vi "Review Fiducials Dialog.vi"(7 "Console Log in":refnum<class "Console Log.lvclass">, 8 "error in":errorcluster, 11 "Potting Procedure in":refnum<class "Potting Procedure.lvclass">) -> (0 "error out":errorcluster, 2 "Canceled":bool, 3 "Potting Procedure out":refnum<class "Potting Procedure.lvclass">, 5 "Console Log out":refnum<class "Console Log.lvclass">)   [LabVIEW 2011]
uses:
  Procedure Classes/Potting Procedure/Potting Procedure.lvclass
  UI Classes/Console Log/Console Log.lvclass
  Shared Components/Utils/Type Definitions/Fiducial with Source.ctl
  Shared Components/Vec3d Class/Vec3d Class.lvclass
  Procedure Classes/Potting Procedure/Type Definitions/Inspect Fiducials.ctl
  Shared Components/Utils/Type Definitions/Fiducial Image.ctl
  Shared Components/Utils/Type Definitions/Physical Image.ctl
  <vilib>/vision/Image Controls.llb/IMAQ Image.ctl
  Procedure Classes/Potting Procedure/Type Definitions/Review Fiducials.ctl
panel:
  out "BBM BL View":T1(plugin-control)
  out "BBM BR View":T1(plugin-control)
  out "BBM TL View":T1(plugin-control)
  out "BBM TR View":T1(plugin-control)
  in  "idx":i32
  out "idx_label":string="1/10"
  out "Current Module":cluster{"Chuck":i32, "Slot":i32}={"Chuck"=1, "Slot"=1}
  in  "Previous":bool
  in  "Next":bool
  out "HDI BL View":T1(plugin-control)
  out "HDI BR View":T1(plugin-control)
  out "HDI TL View":T1(plugin-control)
  out "HDI TR View":T1(plugin-control)
  in  "OK Button":bool
  in  "Cancel Button":bool
  # "Pattern Recognition"
  # "Error"
  # "Click on images to correct fiducial positions.\nAll error fiducials must be corrected before continuing."
  # "User Defined"
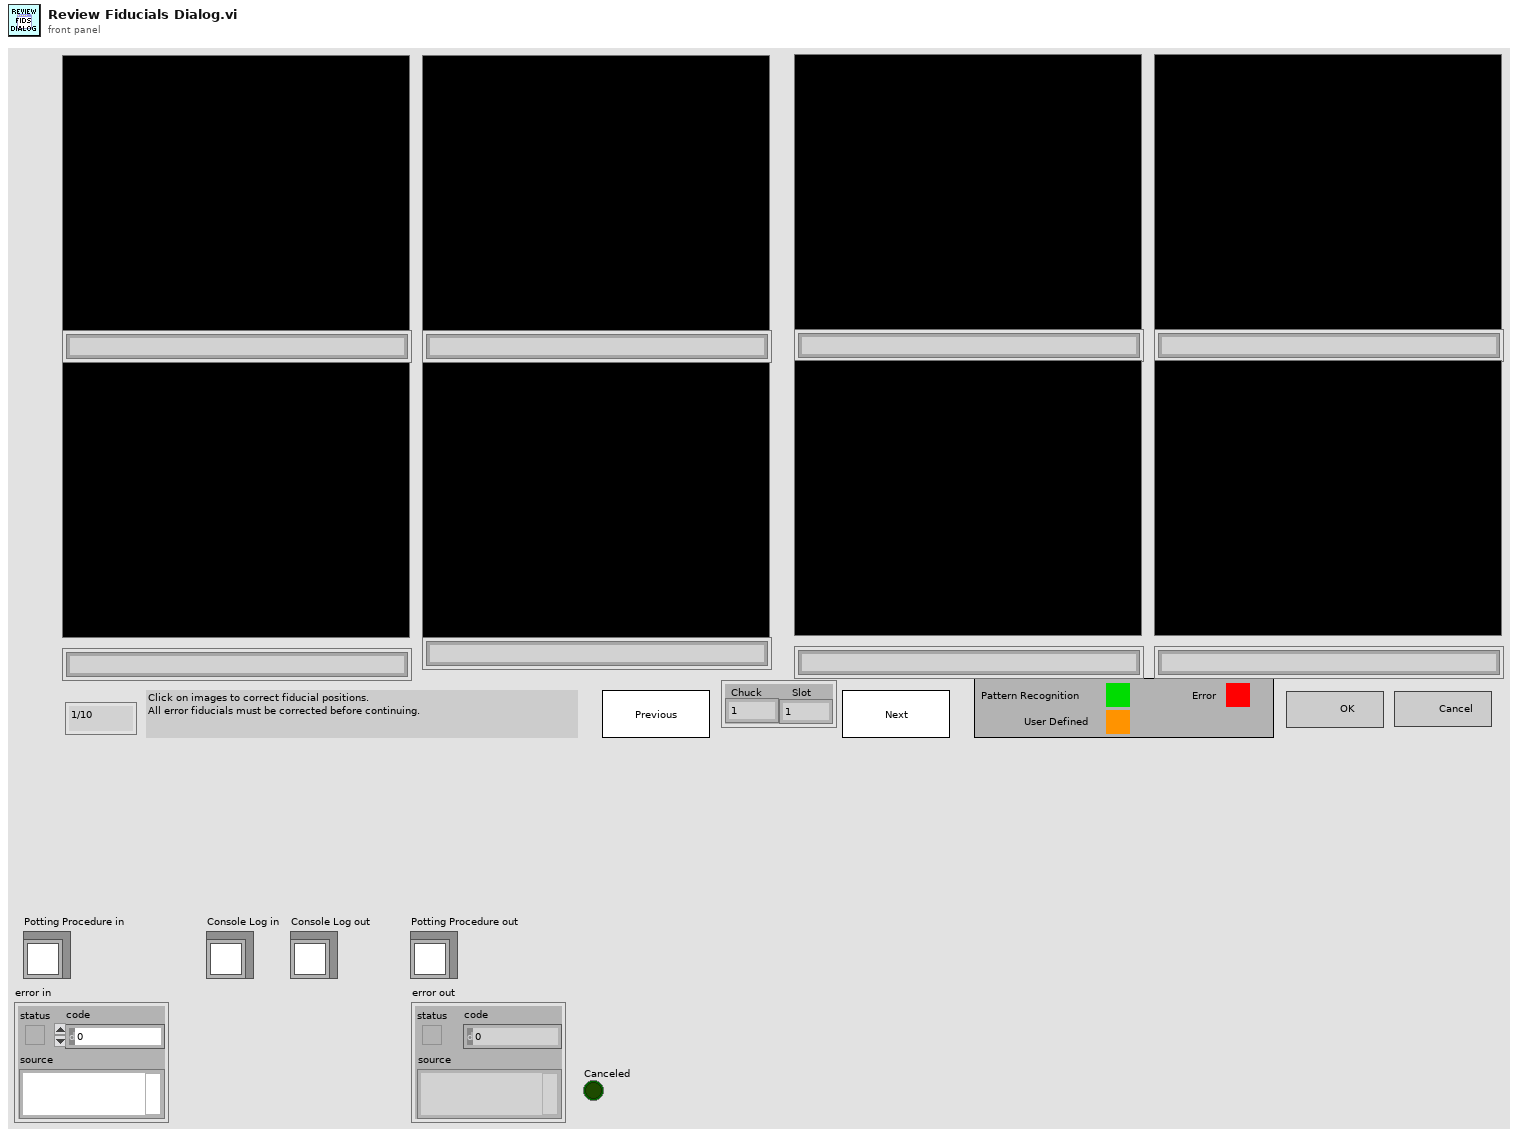
[diagram p1: front panel]
types:
  T1 = typedef "IMAQ Image.ctl" = refnum<image>
  T2 = typedef "Inspect Fiducials.ctl" = cluster{"Has Been Run?":bool, "Module-Chuck Fiducials":cluster{"Fiducials-HDI":T3[], "Fiducials-BBM":T3[], "Chuck":i32, "Slot":i32}[]}
  T3 = typedef "Fiducial Image.ctl" = cluster{"Fiducial Image":T4, "Selected Fiducial":T5, "fiducial name":string}
  T4 = typedef "Physical Image.ctl" = cluster{"Image Position":refnum<class "Vec3d Class.lvclass">, "Image Reference":T1, "Field of View":cluster{"x(mm)":dbl, "y(mm)":dbl}}
  T5 = typedef "Fiducial with Source.ctl" = cluster{"Fiducial Image Coordinate":refnum<class "Vec3d Class.lvclass">, "Fiducial Source":enum16{"Pattern Recognition", "User", "Error", "Default"}}
  T6 = cluster{"Fiducials-HDI":T3[], "Fiducials-BBM":T3[], "Chuck":i32, "Slot":i32}[]
  T7 = cluster{"Fiducials-HDI":T3[], "Fiducials-BBM":T3[], "Chuck":i32, "Slot":i32}
  T8 = enum16{"Pattern Recognition", "User", "Error", "Default"}
  T9 = typedef "LVPoint32TypeDef.ctl" = cluster{"Horizontal":i32, "Vertical":i32}
  T10 = typedef "Review Fiducials.ctl" = cluster{"Has Been Run?":bool}
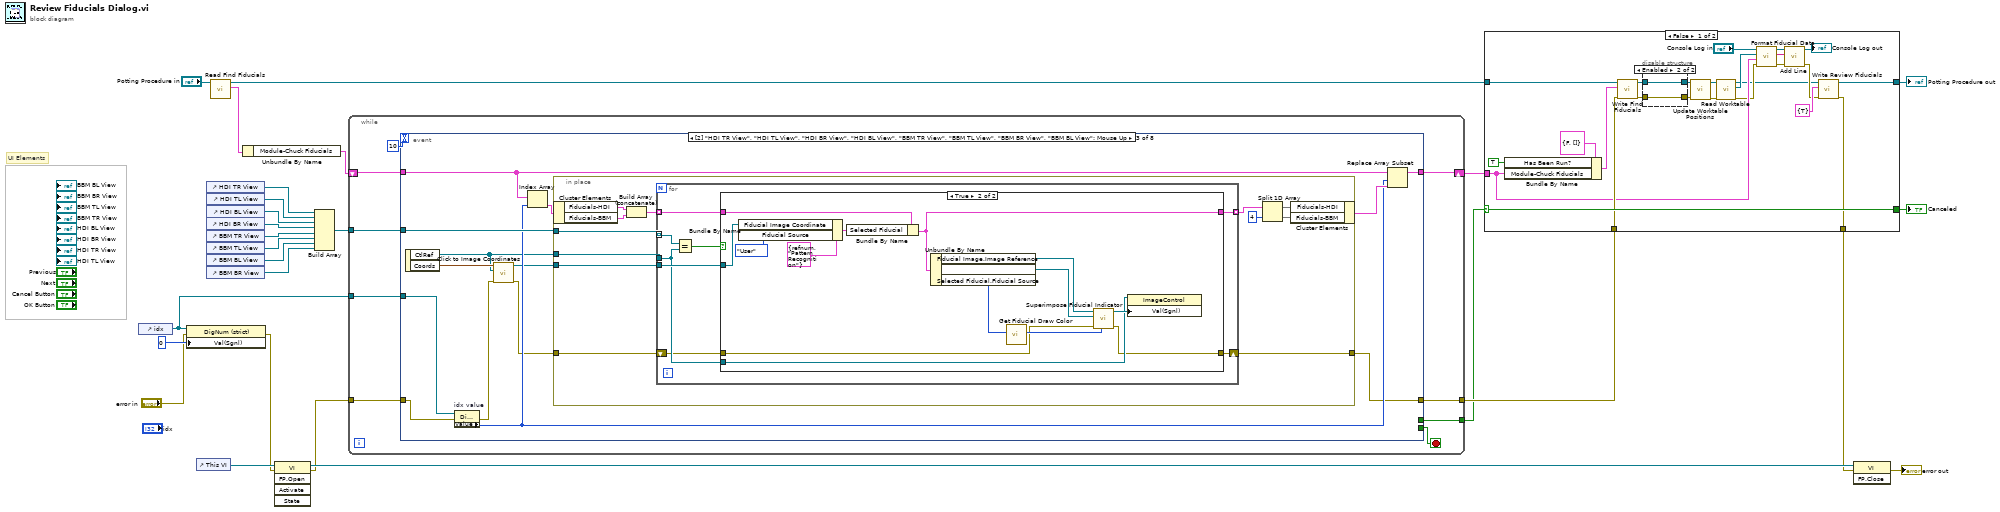
[diagram p0: block diagram]
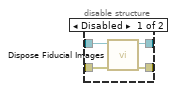
[diagram p2: hidden frame]
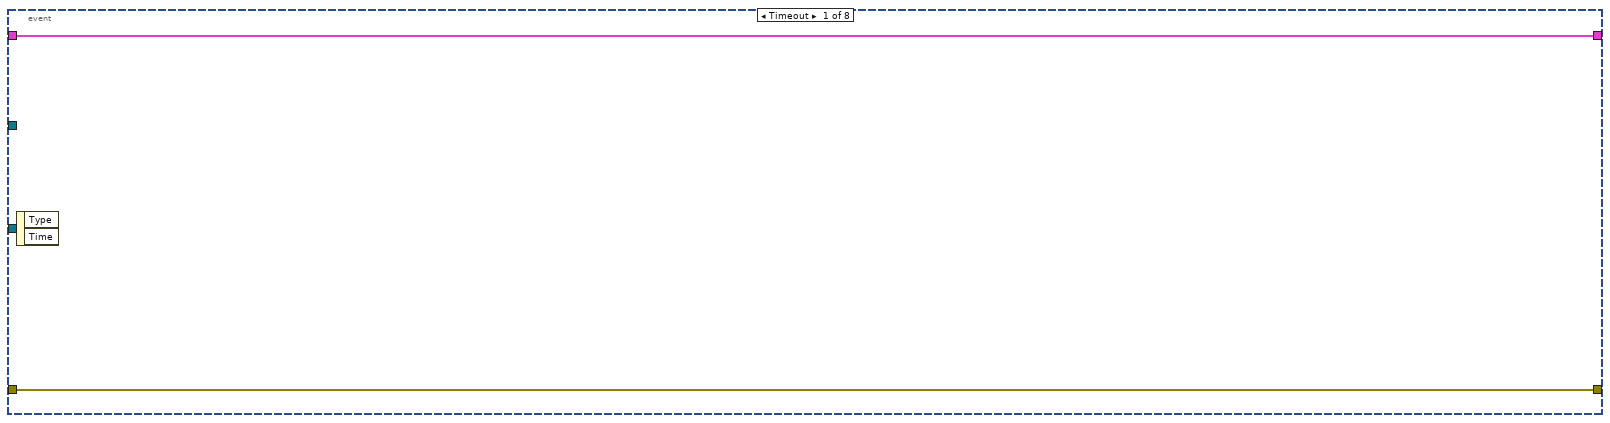
[diagram p4: hidden frame]
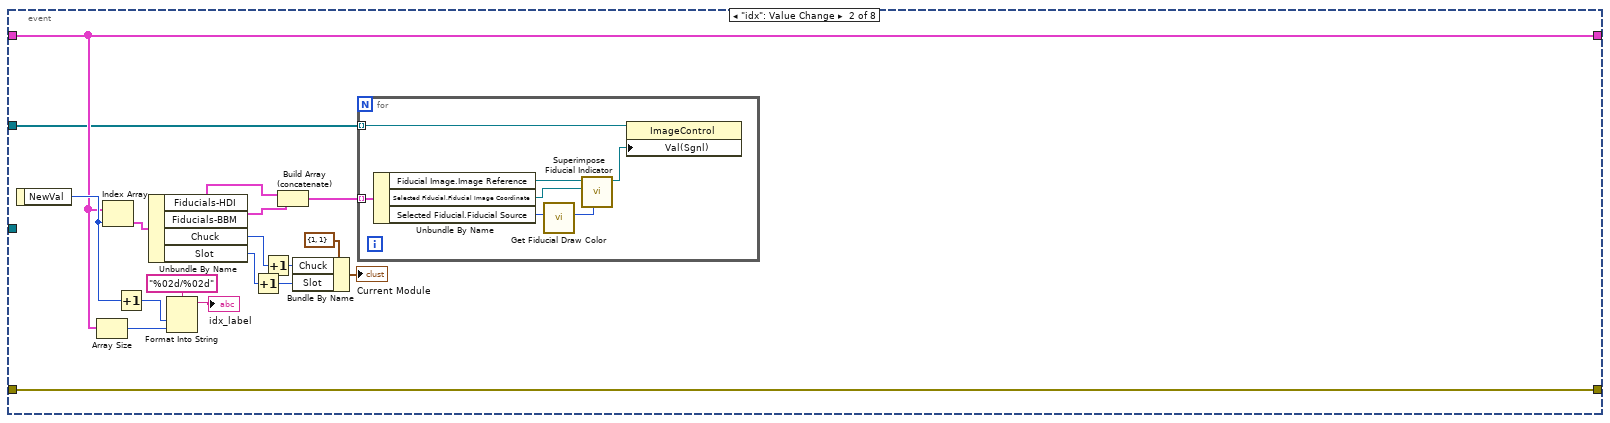
[diagram p5: hidden frame]
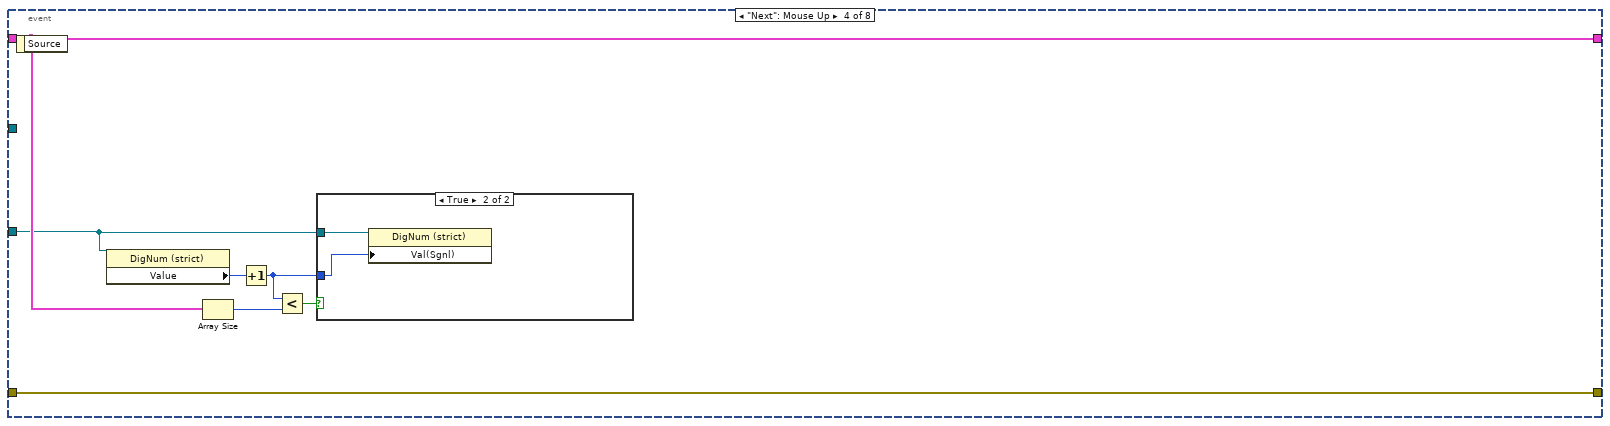
[diagram p7: hidden frame]
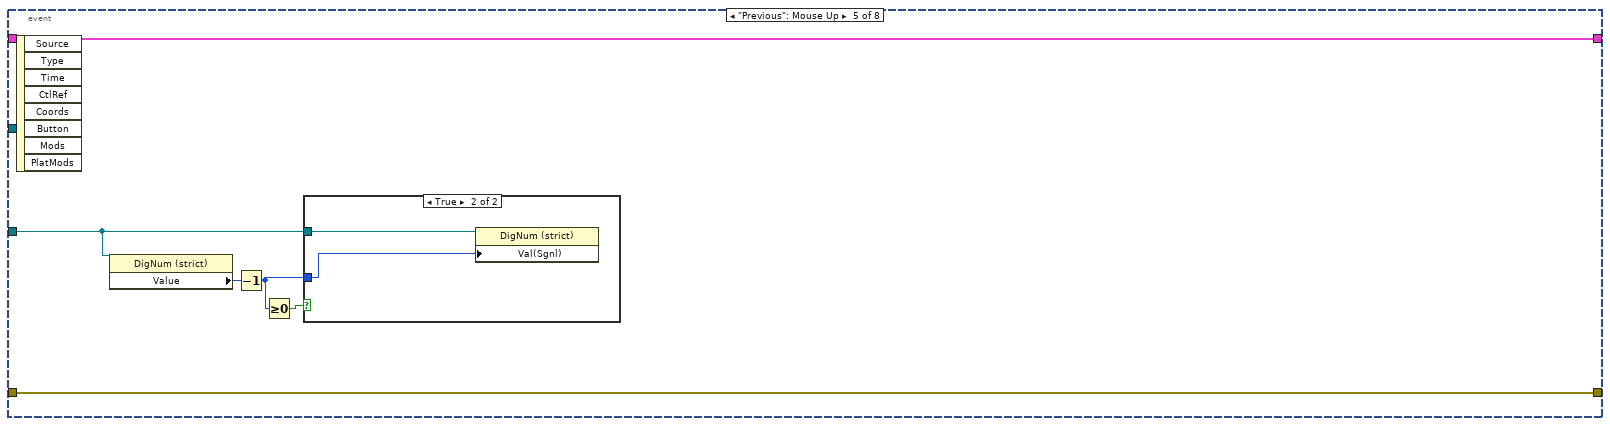
[diagram p9: hidden frame]
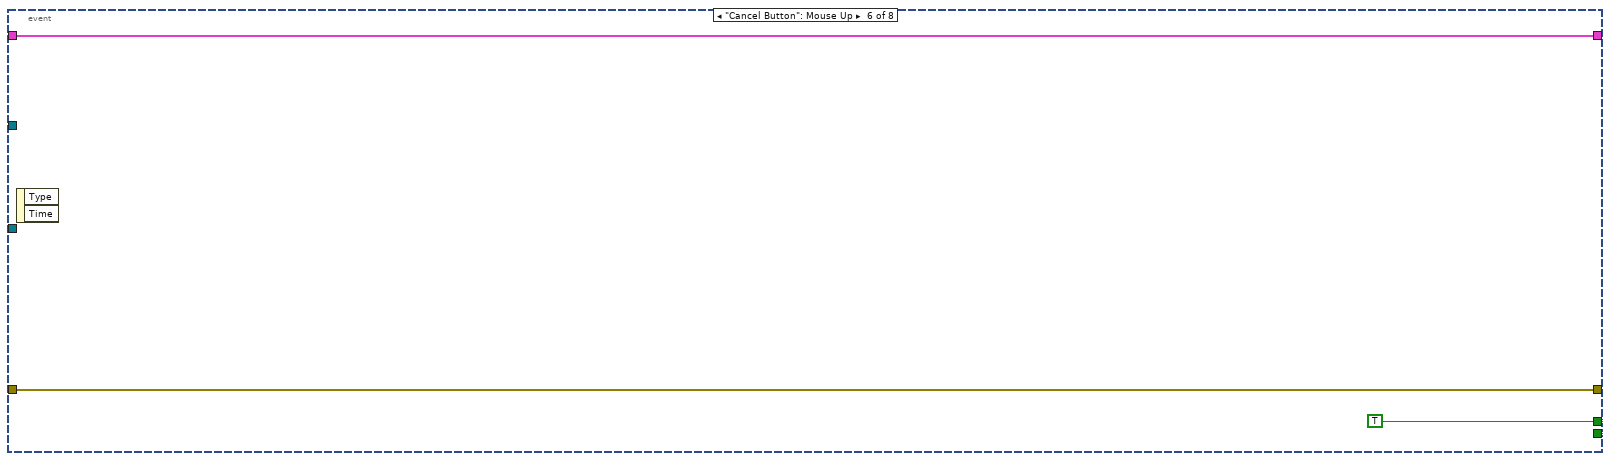
[diagram p11: hidden frame]
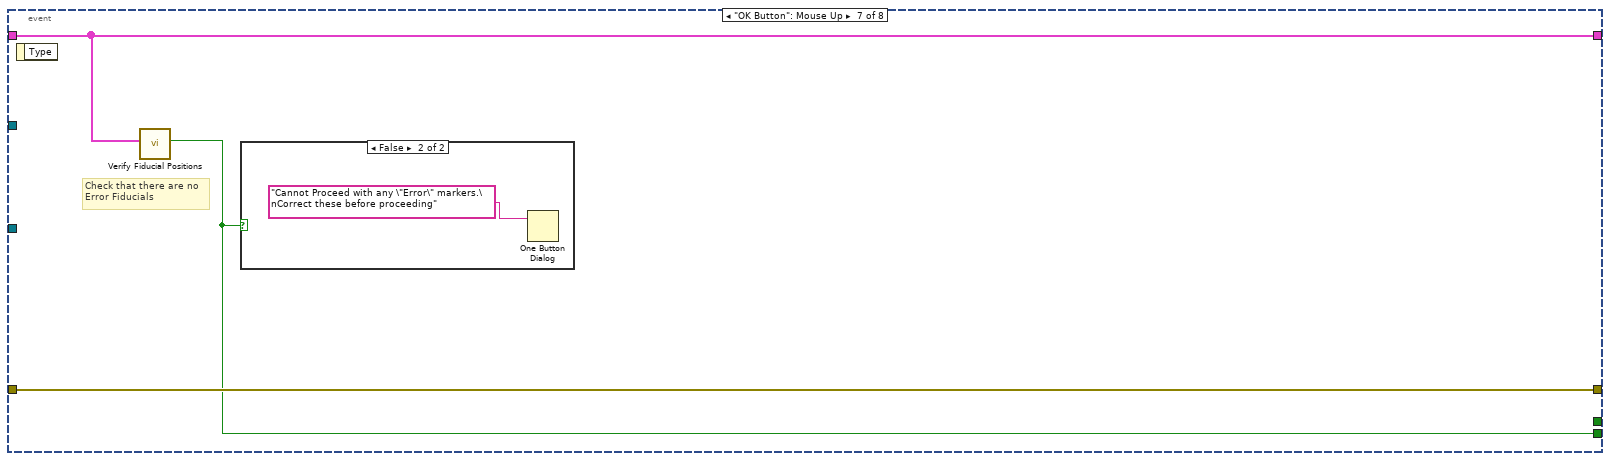
[diagram p12: hidden frame]
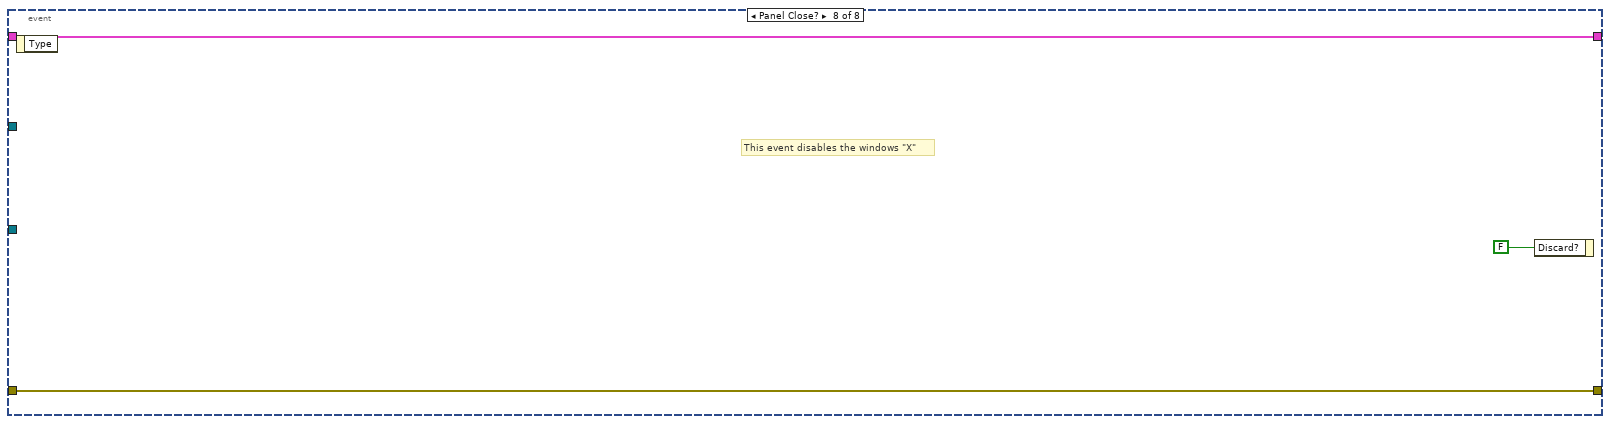
[diagram p14: hidden frame]
diagram:
  # "UI Elements"
  n1 = control-ref of="idx"() -> (w1:refnum<vi>)
  n2 = property class="DigNum (strict)"(reference=w1, error in="error in", "Val(Sgnl)"=0 ("Value (Signaling)")) -> (error out=w9:errorcluster)  [unwired: 1 out]
  n3 = control-ref of="This VI"() -> (w27:refnum<vi>)
  n4 = control-ref of="HDI TR View"() -> (w20:refnum<vi>)
  n5 = control-ref of="HDI TL View"() -> (w19:refnum<vi>)
  n6 = control-ref of="HDI BL View"() -> (w18:refnum<vi>)
  n7 = control-ref of="HDI BR View"() -> (w17:refnum<vi>)
  n8 = control-ref of="BBM TR View"() -> (w16:refnum<vi>)
  n9 = control-ref of="BBM TL View"() -> (w15:refnum<vi>)
  n10 = control-ref of="BBM BL View"() -> (w14:refnum<vi>)
  n11 = control-ref of="BBM BR View"() -> (w13:refnum<vi>)
  n12 = call-dynamic "Read Find Fiducials.vi"("Potting Procedure in"="Potting Procedure in") -> ("Find Fiducials"=w22:T2, "Potting Procedure out"=w5:refnum<class "Potting Procedure.lvclass">)  [unwired: 8 in, 1 out]
  n13 = Unbundle By Name(w22) -> ("Module-Chuck Fiducials"=w21:T6)
  n14 = invoke class="VI" method="FP.Open"(reference=w27, error in=w9) -> (reference out=w26:refnum<vi>, error out=w24:errorcluster)  [unwired: 3 in, 3 out]
  n15 = Build Array(w20, w19, w18, w17, w16, w15, w14, w13) -> (w12:refnum<vi>[])
  n16 = while {
    tunnel: [w32] -> w7
    tunnel: w24 -> [w33]
    tunnel: [w34] -> w8
    shift-right: [w31] -> w6
    shift-left: w21 -> [w30]
    tunnel: w12 -> [w29]
    tunnel: w1 -> [w28]
    stop <- w35 stop-if-true
    n17 = event shown="[2] \"HDI TR View\", \"HDI TL View\", \"HDI BR View\", \"HDI BL View\", \"BBM TR View\", \"BBM TL View\", \"BBM BR View\", \"BBM BL View\": Mouse Up" {
      selector: _ -> [_ _ _ _ _ _ _ _]
      dyn-events: _ -> [_ _ _ _ _ _ _ _]
      timeout: 10 -> [_ _ _ _ _ _ _ _]
      tunnel: [_ _ _ _ _ w132 w134 _] -> w35
      tunnel: [w38 w39 w64 w114 w123 w133 w136 w139] -> w34
      tunnel: w33 -> [w38 w39 w67 w114 w123 w133 w136 w139]
      tunnel: [_ _ _ _ _ w132 _ _] -> w32
      tunnel: [w37 w48 w75 w116 w125 w131 w135 w138] -> w31
      tunnel: w30 -> [w37 w48 w76 w116 w125 w131 w135 w138]
      tunnel: w29 -> [_ w45 w77 _ _ _ _ _]
      tunnel: w28 -> [_ _ w71 w115 w124 _ _ _]
      event Timeout {
        n18 = event-data() -> ()  [unwired: 1 in, 2 out]
      }
      event "idx": Value Change {
        n19 = event-data() -> ("NewVal"=w50:i32)  [unwired: 1 in]
        n20 = Array Size(array=w48) -> (size(s)=w51:i32)
        n21 = Index Array(array=w48, index=w50) -> (element=w56:T7)
        n22 = Increment(x=w50) -> (x+1=w52:i32)
        n23 = Unbundle By Name(w56) -> ("Fiducials-HDI"=w46:T3[], "Fiducials-BBM"=w47:T3[], "Chuck"=w40:i32, "Slot"=w42:i32)
        n24 = Format Into String(format string="%02d/%02d", w52, w51) -> (resulting string=→"idx_label":string)  [unwired: 2 in, 1 out]
        n25 = Increment(x=w42) -> (x+1=w43:i32)
        n26 = Increment(x=w40) -> (x+1=w41:i32)
        n27 = Build Array (concatenate)(w46, w47) -> (w44:T3[])
        n28 = Bundle By Name(cluster=cluster{"Chuck":i32, "Slot":i32} {"Chuck"=1, "Slot"=1} ("Current Module"), "Chuck"=w41, "Slot"=w43) -> (→"Current Module":cluster{"Chuck":i32, "Slot":i32})
        n29 = for {
          tunnel: w45 -> [w62] mode=indexing
          tunnel: w44 -> [w63] mode=indexing
          n30 = Unbundle By Name(w63) -> ("Fiducial Image.Image Reference"=w61:T1, "Selected Fiducial.Fiducial Image Coordinate"=w59:refnum<class "Vec3d Class.lvclass">, "Selected Fiducial.Fiducial Source"=w58:T8)
          n31 = call "Get Fiducial Draw Color.vi"("Fiducial Source"=w58) -> ("Grid Line Color"=w57:u32)  [unwired: 10 in]
          n32 = call "Superimpose Fiducial Indicator.vi"("Marker Color"=w57, "Fiducial Image Coordinates"=w59, "Image In"=w61) -> ("Image Out"=w60:T1)  [unwired: 7 in, 1 out]
          n33 = property class="ImageControl"(reference=w62, "Val(Sgnl)"=w60) -> ()  [unwired: 1 in, 2 out]
        }
      }
      event "HDI TR View", "HDI TL View", "HDI BR View", "HDI BL View", "BBM TR View", "BBM TL View", "BBM BR View", "BBM BL View": Mouse Up {
        n34 = event-data() -> ("CtlRef"=w68:refnum<vi>, "Coords"=w69:T9)  [unwired: 1 in]
        n35 = property on="idx value" class="DigNum (strict)"(reference=w71, error in=w67) -> (error out=w66:errorcluster, "Value"=w72:i32)  [unwired: 1 out]
        n36 = call "Click to Image Coordinates.vi"("error in"=w66, "Display Reference"=w68, "Coords"=w69) -> ("error out"=w65:errorcluster, "Image Coordinates"=w70:refnum<class "Vec3d Class.lvclass">)  [unwired: 7 in]
        n37 = Index Array(array=w76, index=w72) -> (element=w74:T7)
        n38 = in-place {
          in-place-border: w77 -> [w89]
          in-place-border: w68 -> [w87]
          in-place-border: w70 -> [w86]
          in-place-border: w65 -> [w79]
          in-place-border: [w78] -> w64
          n39 = in-place-cluster #1(w74) -> ("Fiducials-HDI"=w85:T3[], "Fiducials-BBM"=w84:T3[])
          n40 = Build Array (concatenate)(w85, w84) -> (w88:T3[])
          n41 = for {
            tunnel: w89 -> [w95] mode=indexing
            tunnel: w88 -> [w97] mode=indexing
            tunnel: w87 -> [w92]
            tunnel: w86 -> [w94]
            tunnel: [w93] -> w83 mode=indexing
            shift-right: [w90] -> w78
            shift-left: w79 -> [w91]
            n42 = Equal?(x=w95, y=w92) -> (x = y?=w96:bool)
            n43 = case shown="True" w96 {
              tunnel: w97 -> [w99 w109]
              tunnel: w94 -> [_ w112]
              tunnel: [w99 w105] -> w93
              tunnel: w92 -> [_ w104]
              tunnel: w91 -> [w98 w101]
              tunnel: [w98 w100] -> w90
              frame False {
              }
              frame True {
                n44 = Bundle By Name(cluster=T5 {"Fiducial Image Coordinate"=refnum, "Fiducial Source"=enum."Pattern Recognition"} ("Selected Fiducial"), "Fiducial Image Coordinate"=w112, "Fiducial Source"=enum16{"Pattern Recognition", "User", "Error"}."User") -> (w110:T5)
                n45 = Bundle By Name(cluster=w109, "Selected Fiducial"=w110) -> (w105:T3)
                n46 = Unbundle By Name(w105) -> ("Fiducial Image.Image Reference"=w107:T1, "Selected Fiducial.Fiducial Image Coordinate"=w106:refnum<class "Vec3d Class.lvclass">, "Selected Fiducial.Fiducial Source"=w103:T8)
                n47 = call "Get Fiducial Draw Color.vi"("Fiducial Source"=w103) -> ("Grid Line Color"=w102:u32)  [unwired: 10 in]
                n48 = call "Superimpose Fiducial Indicator.vi"("Marker Color"=w102, "error in"=w101, "Fiducial Image Coordinates"=w106, "Image In"=w107) -> ("error out"=w100:errorcluster, "Image Out"=w108:T1)  [unwired: 6 in]
                n49 = property class="ImageControl"(reference=w104, "Val(Sgnl)"=w108) -> ()  [unwired: 1 in, 2 out]
              }
            }
          }
          n50 = Split 1D Array(array=w83, index=4) -> (first subarray=w82:T3[], second subarray=w81:T3[])
          n51 = in-place-cluster #1("Fiducials-HDI"=w82, "Fiducials-BBM"=w81) -> (w73:T7)
        }
        n52 = Replace Array Subset(array=w76, new element=w73, index=w72) -> (w75:T6)
      }
      event "Next": Mouse Up {
        n53 = event-data() -> ()  [unwired: 1 in, 1 out]
        n54 = property class="DigNum (strict)"(reference=w115) -> ("Value"=w120:i32)  [unwired: 1 in, 2 out]
        n55 = Array Size(array=w116) -> (size(s)=w119:i32)
        n56 = Increment(x=w120) -> (x+1=w117:i32)
        n57 = Less?(x=w117, y=w119) -> (x < y?=w118:bool)
        n58 = case shown="True" w118 {
          tunnel: w117 -> [_ w121]
          tunnel: w115 -> [_ w122]
          frame False {
          }
          frame True {
            n59 = property class="DigNum (strict)"(reference=w122, "Val(Sgnl)"=w121) -> ()  [unwired: 1 in, 2 out]
          }
        }
      }
      event "Previous": Mouse Up {
        n60 = event-data() -> ()  [unwired: 1 in, 8 out]
        n61 = property class="DigNum (strict)"(reference=w124) -> ("Value"=w128:i32)  [unwired: 1 in, 2 out]
        n62 = Decrement(x=w128) -> (x-1=w126:i32)
        n63 = Greater Or Equal To 0?(x=w126) -> (x >= 0?=w127:bool)
        n64 = case shown="True" w127 {
          tunnel: w126 -> [_ w129]
          tunnel: w124 -> [_ w130]
          frame False {
          }
          frame True {
            n65 = property class="DigNum (strict)"(reference=w130, "Val(Sgnl)"=w129) -> ()  [unwired: 1 in, 2 out]
          }
        }
      }
      event "Cancel Button": Mouse Up {
        w132 = TRUE
        n66 = event-data() -> ()  [unwired: 1 in, 2 out]
      }
      event "OK Button": Mouse Up {
        # "Check that there are no\nError Fiducials"
        n67 = event-data() -> ()  [unwired: 1 in, 1 out]
        n68 = call "Verify Fiducial Positions.vi"("Module Fiducials"=w135) -> ("All Good"=w134:bool)  [unwired: 9 in, 1 out]
        n69 = case shown="False" w134 {
          frame True {
          }
          frame False {
            n70 = One Button Dialog(message="Cannot Proceed with any \"Error\" markers.\nCorrect these before proceeding") -> ()  [unwired: 1 in, 1 out]
          }
        }
      }
      event Panel Close? {
        # "This event disables the windows \"X\""
        n71 = event-data() -> ()  [unwired: 1 in, 1 out]
        n72 = event-data("Discard?"=FALSE) -> ()  [unwired: 1 in, 1 out]
      }
    }
  }
  n73 = case shown="False" w7 {
    selector: w7 -> [w165 w172]
    tunnel: w8 -> [w162 w173]
    tunnel: w6 -> [w148 _]
    tunnel: w5 -> [w157 w174]
    tunnel: [w164 w174] -> w4
    tunnel: [w161 w173] -> w3
    tunnel: [w165 w172] -> w2
    frame False {
      n74 = Bundle By Name(cluster=T2 {"Has Been Run?"=FALSE, "Module-Chuck Fiducials"=[]} ("Find Fiducials"), "Has Been Run?"=TRUE, "Module-Chuck Fiducials"=w148) -> (w158:T2)
      n75 = call-dynamic "Write Find Fiducials.vi"("error in"=w162, "Find Fiducials"=w158, "Potting Procedure in"=w157) -> ("error out"=w154:errorcluster, "Potting Procedure out"=w156:refnum<class "Potting Procedure.lvclass">)  [unwired: 7 in]
      n76 = disable-structure shown="Enabled" {
        disable-tunnel: w156 -> [w169 w171]
        disable-tunnel: [w168 w171] -> w155
        disable-tunnel: w154 -> [w167 w170]
        disable-tunnel: [w166 w170] -> w153
        frame Disabled {
          n77 = call-dynamic "Dispose Fiducial Images.vi"("error in"=w167, "Potting Procedure in"=w169) -> ("error out"=w166:errorcluster, "Potting Procedure out"=w168:refnum<class "Potting Procedure.lvclass">)  [unwired: 8 in]
        }
        frame Enabled {
        }
      }
      n78 = call-dynamic "Update Worktable Positions.vi"("error in"=w153, "Potting Procedure in"=w155) -> ("error out"=w151:errorcluster, "Potting Procedure out"=w152:refnum<class "Potting Procedure.lvclass">)  [unwired: 8 in]
      n79 = call-dynamic "Read Worktable.vi"("error in"=w151, "Potting Procedure in"=w152) -> ("error out"=w144:errorcluster, "WorkTable out"=w149:refnum<class "WorkTable Class.lvclass">, "Potting Procedure out"=w141:refnum<class "Potting Procedure.lvclass">)  [unwired: 7 in]
      n80 = call "Format Fiducial Data.vi"("error in"=w144, "Module-Chuck Fiducials"=w148, "Worktable"=w149, "Console Log in"="Console Log in") -> ("error out"=w143:errorcluster, "Formatted Fiducial Data"=w145:string, "Console Log out"=w147:refnum<class "Console Log.lvclass">)  [unwired: 5 in]
      n81 = call "Add Line.vi"("error in"=w143, "String"=w145, "Console Log in"=w147) -> ("error out"=w142:errorcluster, "Console Log out"=→"Console Log out":refnum<class "Console Log.lvclass">)  [unwired: 7 in]
      n82 = call-dynamic "Write Review Fiducials.vi"("error in (no error)"=w142, "Review Fiducials"=T10 {"Has Been Run?"=TRUE}, "Potting Procedure in"=w141) -> ("error out"=w161:errorcluster, "Potting Procedure out"=w164:refnum<class "Potting Procedure.lvclass">)  [unwired: 7 in]
    }
    frame True {
    }
  }
  "Canceled" <- w2
  "Potting Procedure out" <- w4
  n83 = invoke class="VI" method="FP.Close"(reference=w26, error in=w3) -> (error out=→"error out":errorcluster)  [unwired: 1 in, 2 out]
